vi "callResponse.vi"(3 "error in (no error)":errorcluster, 4 "input":u8[](array[numeric]), 5 "TCP Network Connection in":refnum<k5>) -> (0 "error out":errorcluster, 1 "unsigned byte array":u8[](array[numeric]), 2 "TCP Network Connection out":refnum<k5>)   [LabVIEW 2021]
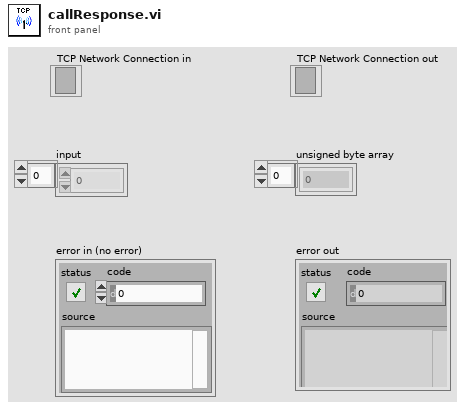
[diagram p1: front panel]
types:
  T1 = enum16{"big-endian, network order", "native, host order", "little-endian"}
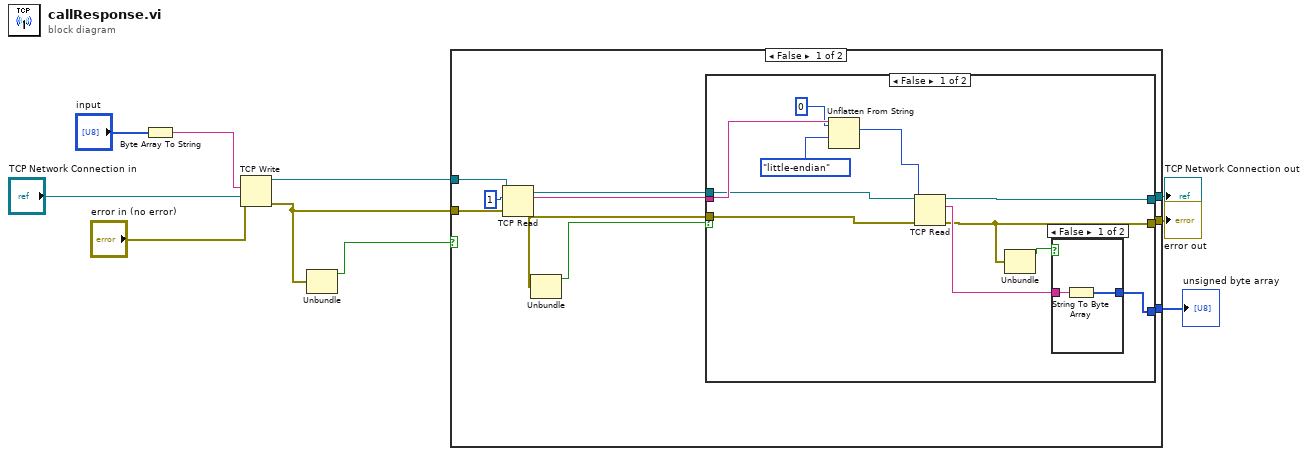
[diagram p0: block diagram]
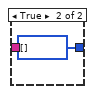
[diagram p2: hidden frame]
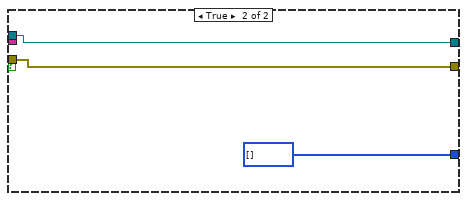
[diagram p3: hidden frame]
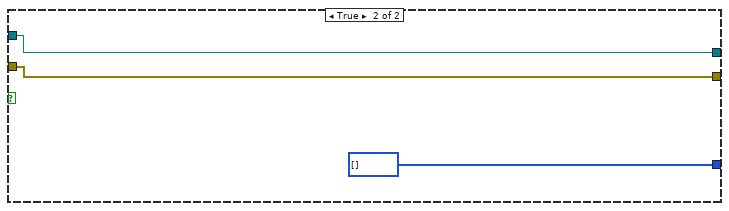
[diagram p4: hidden frame]
diagram:
  n1 = Byte Array To String(unsigned byte array="input") -> (string=w3:string)
  n2 = TCP Write(connection ID="TCP Network Connection in", data in=w3, error in (no error)="error in (no error)") -> (connection ID out=w7:refnum<k5>, error out=w2:errorcluster)  [unwired: 1 in, 1 out]
  n3 = Unbundle(w2) -> ("status"=w1:bool)  [unwired: 2 out]
  n4 = case shown="False" w1 {
    tunnel: [w19 u8[] [] ("unsigned byte array")] -> w10
    tunnel: [w18 w39] -> w9
    tunnel: [w17 w40] -> w8
    tunnel: w7 -> [w16 w40]
    tunnel: w2 -> [w12 w39]
    frame False {
      n5 = TCP Read(connection ID=w16, bytes to read=1, error in (no error)=w12) -> (connection ID out=w15:refnum<k5>, data out=w20:string, error out=w13:errorcluster)  [unwired: 2 in]
      n6 = Unbundle(w13) -> ("status"=w11:bool)  [unwired: 2 out]
      n7 = case shown="False" w11 {
        tunnel: w20 -> [w30 _]
        tunnel: [w29 u8[] [] ("unsigned byte array")] -> w19
        tunnel: [w22 w36] -> w18
        tunnel: [w28 w37] -> w17
        tunnel: w15 -> [w26 w37]
        tunnel: w13 -> [w23 w36]
        frame False {
          n8 = Unflatten From String(type=u8 0, binary string=w30, byte order (0:big-endian, network order)=T1."little-endian") -> (value=w31:u8)  [unwired: 2 in, 2 out]
          n9 = TCP Read(connection ID=w26, bytes to read=w31, error in (no error)=w23) -> (connection ID out=w28:refnum<k5>, data out=w27:string, error out=w22:errorcluster)  [unwired: 2 in]
          n10 = Unbundle(w22) -> ("status"=w21:bool)  [unwired: 2 out]
          n11 = case shown="False" w21 {
            tunnel: [w33 u8[] [] ("unsigned byte array")] -> w29
            tunnel: w27 -> [w32 _]
            frame False {
              n12 = String To Byte Array(string=w32) -> (unsigned byte array=w33:u8[])
            }
            frame True {
            }
          }
        }
        frame True {
        }
      }
    }
    frame True {
    }
  }
  "unsigned byte array" <- w10
  "error out" <- w9
  "TCP Network Connection out" <- w8
